vi "Simulator.vi"(8 "error in":errorcluster) -> (0 "error out":errorcluster, 2 "FFT":cluster{"f0":dbl, "df":dbl, "magnitude":dbl[]}[](array[cluster]), 3 "Wave":waveform(dbl)[](array[waveform]))   [LabVIEW 2018]
uses:
  <vilib>/measure/maspectr.llb/FFT Power Spectrum and PSD for 1 Chan.vi
  <vilib>/measure/NI_MABase.lvlib
  <vilib>/measure/NI_MAPro.lvlib
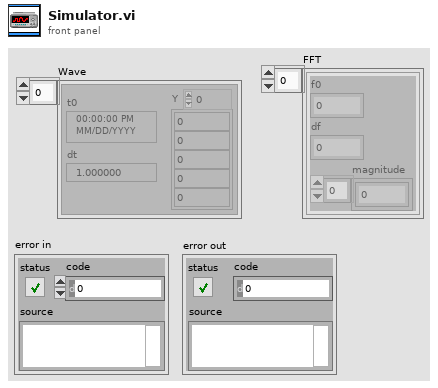
[diagram p1: front panel]
types:
  T1 = enum16{"Save File", "Read File", "Put Frequency", "Put Signal Type", "Put Channel", "Put All", "Get All"}
  T2 = typedef "Parameter.ctl" = cluster{"Channel Count":T3, "Frequency Setting":T4, "Signal Type Setting":T5}
  T3 = typedef "Channel Count.ctl" = enum32{"1", "2", "3", "4"}
  T4 = typedef "Frequency Setting.ctl" = enum32{"10 Hz", "50 Hz", "100 Hz"}
  T5 = typedef "Signal Type Setting.ctl" = enum32{"Sine", "Sqaure", "Triangle"}
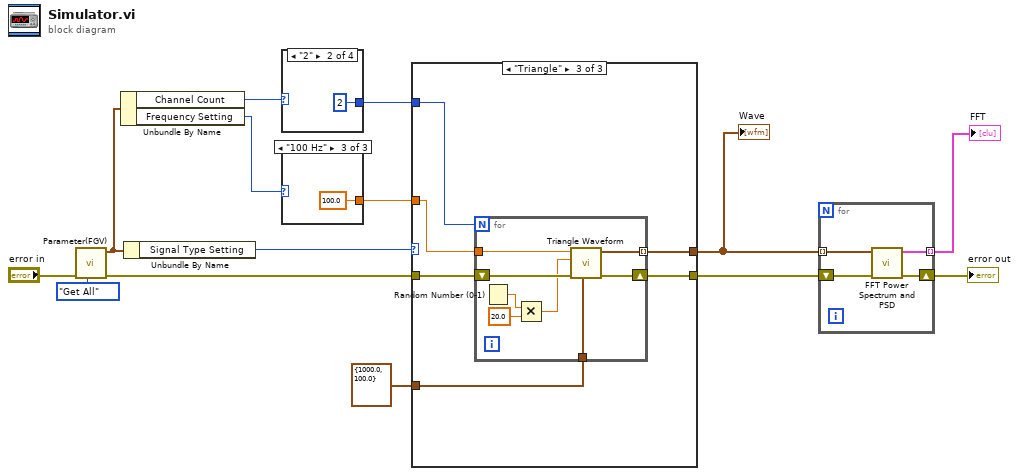
[diagram p0: block diagram]
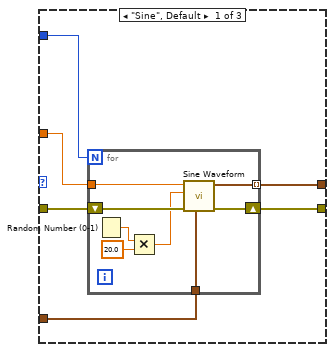
[diagram p2: hidden frame]
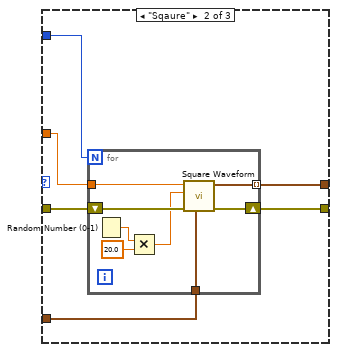
[diagram p3: hidden frame]
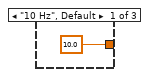
[diagram p4: hidden frame]
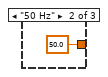
[diagram p5: hidden frame]
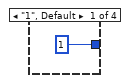
[diagram p6: hidden frame]
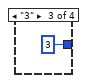
[diagram p7: hidden frame]
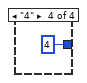
[diagram p8: hidden frame]
diagram:
  n1 = call "Parameter(FGV).vi"("Parameter Method"=T1."Get All", "error in"="error in") -> ("error out"=w9:errorcluster, "Parameter Out"=w11:T2)  [unwired: 8 in]
  n2 = Unbundle By Name(w11) -> ("Channel Count"=w13:T3, "Frequency Setting"=w12:T4)
  n3 = Unbundle By Name(w11) -> ("Signal Type Setting"=w10:T5)
  n4 = case shown="\"2\"" w13 {
    tunnel: [1 2 3 4] -> w7
    frame "1", Default {
    }
    frame "2" {
    }
    frame "3" {
    }
    frame "4" {
    }
  }
  n5 = case shown="\"100 Hz\"" w12 {
    tunnel: [10.0 ("frequency") 50.0 ("frequency") 100.0 ("frequency")] -> w8
    frame "10 Hz", Default {
    }
    frame "50 Hz" {
    }
    frame "100 Hz" {
    }
  }
  n6 = case shown="\"Triangle\"" w10 {
    tunnel: w9 -> [w27 w41 w55]
    tunnel: w8 -> [w25 w39 w52]
    tunnel: w7 -> [w26 w38 w51]
    tunnel: [w24 w37 w53] -> w2
    tunnel: [w23 w40 w54] -> w6
    tunnel: cluster{"Fs":dbl, "#s":dbl} {"Fs"=1000.0, "#s"=100.0} ("sampling info") -> [w22 w36 w50]
    frame "Sine", Default {
      n7 = for {
        N: w26 -> [_]
        tunnel: w25 -> [w34]
        tunnel: [w30] -> w24 mode=indexing
        shift-right: [w29] -> w23
        shift-left: w27 -> [w35]
        tunnel: w22 -> [w28]
        n8 = Random Number (0-1)() -> (number: 0 to 1=w32:dbl)
        n9 = Multiply(x=w32, y=20.0) -> (x*y=w31:dbl)
        n10 = call <vilib>:"Sine Waveform.vi"("sampling info"=w28, "error in (no error)"=w35, "amplitude"=w31, "frequency"=w34) -> ("error out"=w29:errorcluster, "signal out"=w30:waveform(dbl))  [unwired: 6 in]
      }
    }
    frame "Sqaure" {
      n11 = for {
        N: w38 -> [_]
        tunnel: w39 -> [w48]
        tunnel: [w44] -> w37 mode=indexing
        shift-right: [w43] -> w40
        shift-left: w41 -> [w49]
        tunnel: w36 -> [w42]
        n12 = Random Number (0-1)() -> (number: 0 to 1=w46:dbl)
        n13 = Multiply(x=w46, y=20.0) -> (x*y=w45:dbl)
        n14 = call <vilib>:"Square Waveform.vi"("sampling info"=w42, "error in (no error)"=w49, "amplitude"=w45, "frequency"=w48) -> ("error out"=w43:errorcluster, "signal out"=w44:waveform(dbl))  [unwired: 6 in]
      }
    }
    frame "Triangle" {
      n15 = for {
        N: w51 -> [_]
        tunnel: w52 -> [w62]
        tunnel: [w58] -> w53 mode=indexing
        shift-right: [w57] -> w54
        shift-left: w55 -> [w63]
        tunnel: w50 -> [w56]
        n16 = Random Number (0-1)() -> (number: 0 to 1=w60:dbl)
        n17 = Multiply(x=w60, y=20.0) -> (x*y=w59:dbl)
        n18 = call <vilib>:"Triangle Waveform.vi"("sampling info"=w56, "error in (no error)"=w63, "amplitude"=w59, "frequency"=w62) -> ("error out"=w57:errorcluster, "signal out"=w58:waveform(dbl))  [unwired: 6 in]
      }
    }
  }
  "Wave" <- w2
  n19 = for {
    tunnel: [w67] -> w1 mode=indexing
    tunnel: w2 -> [w65] mode=indexing
    shift-right: [w64] -> w4
    shift-left: w6 -> [w66]
    n20 = call-poly <vilib>:"FFT Power Spectrum and PSD.vi"("error in (no error)"=w66, "time signal"=w65) -> ("error out"=w64:errorcluster, "Power Spectrum / PSD"=w67:cluster{"f0":dbl, "df":dbl, "magnitude":dbl[]})  [unwired: 6 in, 2 out]
  }
  "FFT" <- w1
  "error out" <- w4
